vi "LvFifoVI.vi"() -> ()   [LabVIEW 2023]
uses:
  <vilib>/rvi/DataTransferAndStorage/Container/XNode/niFpgaContainer.xnode
  <vilib>/rvi/interface/RandomDataEmulation/nirviRandomDataFpgaReadWriteTemplate.vi
panel:
  out "WriteTimedOut":bool
  out "ReadTimedOut":bool
  out "Number of Elements to Write":u32
  out "Number of Elements to Read":u32
  out "Numeric":i32
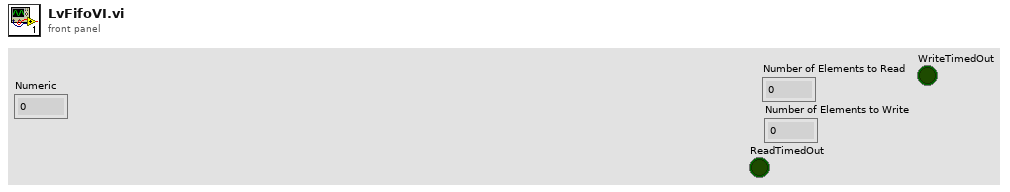
[diagram p1: front panel]
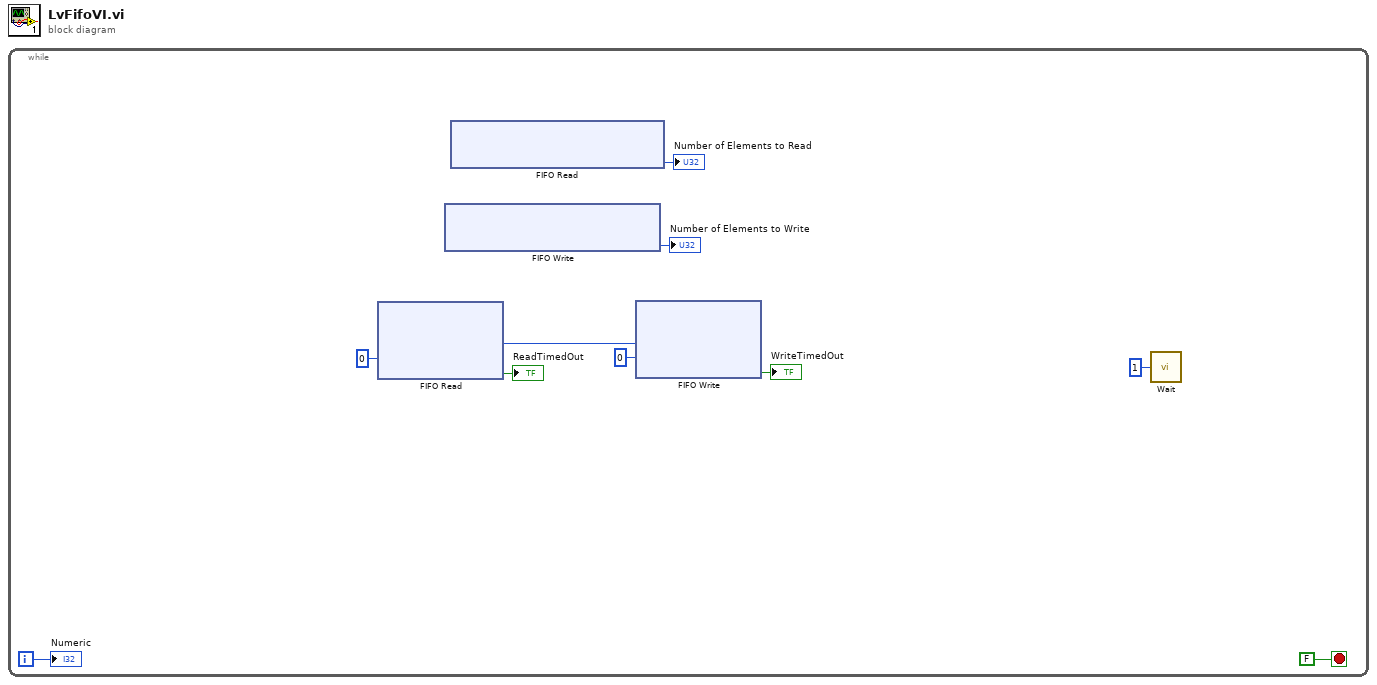
[diagram p0: block diagram]
diagram:
  n1 = while {
    i -> [w9]
    stop <- FALSE stop-if-true
    n2 = xnode ("FIFO Read")("Timeout"=0) -> ("Element"=w6:i16, "Timed Out?"=→"ReadTimedOut":bool)  [unwired: 1 in, 1 out]
    n3 = xnode ("FIFO Write")() -> ("Number of Elements to Write"=→"Number of Elements to Write":u32)  [unwired: 1 in, 1 out]
    n4 = xnode ("FIFO Read")() -> ("Number of Elements to Read"=→"Number of Elements to Read":u32)  [unwired: 1 in, 1 out]
    n5 = xnode ("FIFO Write")("Element"=w6, "Timeout"=0) -> ("Timed Out?"=→"WriteTimedOut":bool)  [unwired: 1 in, 1 out]
    n6 = call "Wait"("Count(mSec)"=u32 1) -> ()  [unwired: 1 out]
    "Numeric" <- w9
  }
